vi "Apex model error handler.vi"(5 "Next state if error":string, 6 "Error codes to ignore (none)":i32[](array[numeric]), 7 "Current state":string, 8 "error in (no error)":errorcluster) -> (0 "error out":errorcluster)   [LabVIEW 2018]
doc: "Does nothing if no error.\n\nIf there is an error, sends it to the designated or default error handling state, whichever is appropriate. Also removes all pending queue elements and sends those to the error handling state as well."
uses:
  Model error handling data.ctl
  Queueing/Model queue data.ctl
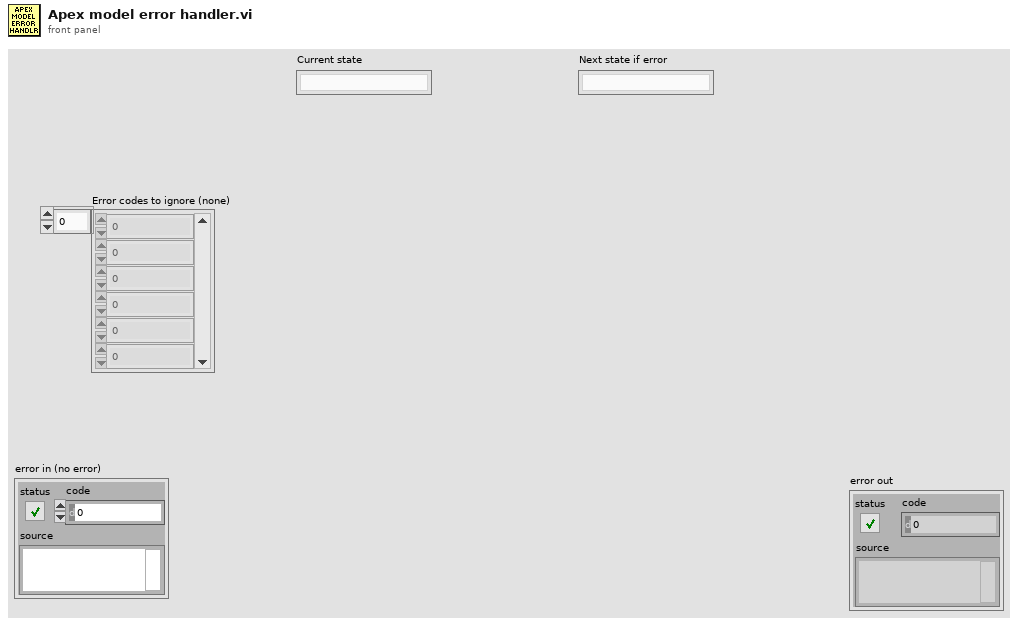
[diagram p1: front panel]
types:
  T1 = typedef "Model error handling data.ctl" = cluster{"Removed queue elements":T2[], "Error to handle":errorcluster, "Originating state":string}
  T2 = typedef "Model queue data.ctl" = cluster{"State":string, "Data":variant, "Next state if error":string}
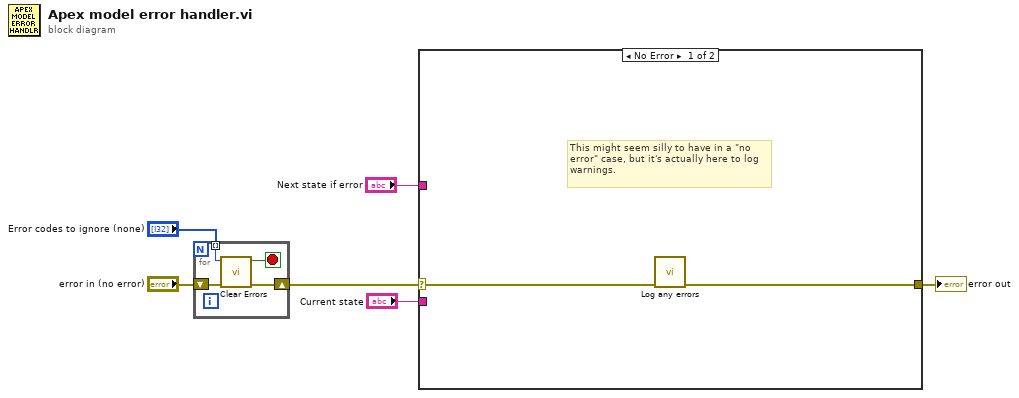
[diagram p0: block diagram]
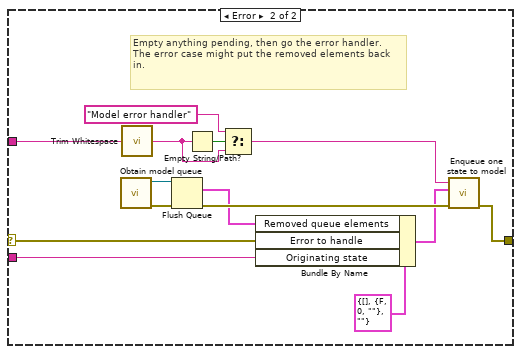
[diagram p2: hidden frame]
diagram:
  n1 = for {
    shift-right: [w9] -> w1
    shift-left: "error in (no error)" -> [w10]
    tunnel: "Error codes to ignore (none)" -> [w8] mode=indexing
    stop <- w7 stop-if-true
    n2 = call <vilib>:"Clear Errors.vi"("error in (no error)"=w10, "specific error code to clear (0: all)"=w8) -> ("error out"=w9:errorcluster, "specific error cleared?"=w7:bool)  [unwired: 4 in]
  }
  n3 = case shown="No Error" w1 {
    selector: w1 -> [w12 w25]
    tunnel: [w11 w22] -> w6
    tunnel: "Next state if error" -> [_ w26]
    tunnel: "Current state" -> [_ w13]
    frame No Error {
      # "This might seem silly to have in a \"no error\" case, but it's actually here to log warnings."
      n4 = call <userlib>:"Log any errors.vi"("error in (no error)"=w12) -> ("error out"=w11:errorcluster)  [unwired: 10 in]
    }
    frame Error {
      # "Empty anything pending, then go the error handler.  The error case might put the removed elements back in."
      n5 = call "Obtain model queue.vi"() -> ("error out"=w24:errorcluster, "Model loop queue"=w23:refnum<queue>)  [unwired: 10 in]
      n6 = call <vilib>:"Trim Whitespace.vi"("string"=w26) -> ("trimmed string"=w15:string)  [unwired: 1 in]
      n7 = Flush Queue(queue=w23, error in (no error)=w24) -> (remaining elements=w20:T2[], error out=w21:errorcluster)  [unwired: 1 out]
      n8 = Empty String/Path?(string/path=w15) -> (empty?=w17:bool)
      n9 = Select(t="Model error handler" ("Enqueued state"), s=w17, f=w15) -> (s? t:f=w14:string)
      n10 = Bundle By Name(cluster=T1 {"Removed queue elements"=[], "Error to handle"={"status"=FALSE, "code"=0, "source"=""}, "Originating state"=""} ("output cluster"), "Removed queue elements"=w20, "Error to handle"=w25, "Originating state"=w13) -> (w19:T1)
      n11 = call "Enqueue one state to model.vi"("error in (no error)"=w21, "Enqueued data"=w19, "Enqueued state"=w14) -> ("error out"=w22:errorcluster)  [unwired: 8 in]
    }
  }
  "error out" <- w6
